vi "zmq proxy.vi"(8 "error in (no error)":errorcluster, 9 "capture_":u32, 10 "backend_":u32, 11 "frontend_":u32) -> (0 "error out":errorcluster, 1 "capture_ out":u32, 2 "backend_ out":u32, 3 "frontend_ out":u32, 5 "function return":i32)   [LabVIEW 2025, in "libzmq-v143-mt-4_3_6.lvlib"]
doc: "ZMQ_EXPORT int zmq_proxy (void *frontend_, void *backend_, void *capture_);"
uses:
  libzmq-v143-mt-4_3_6.lvlib
  LV/LibZMQ/libzmq/lv_x86/bin/Release/libzmq-v143-mt-4_3_6.dll
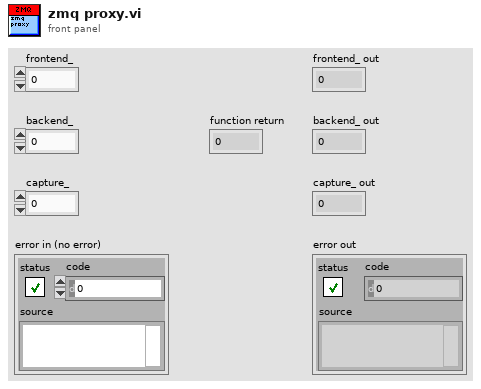
[diagram p1: front panel]
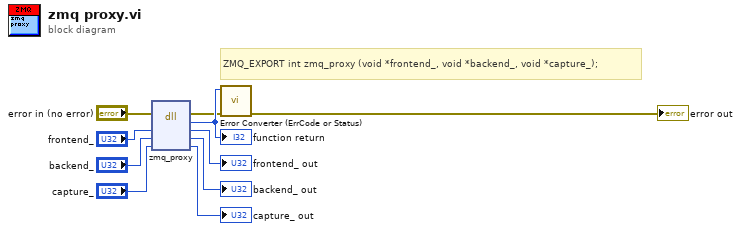
[diagram p0: block diagram]
diagram:
  # "ZMQ_EXPORT int zmq_proxy (void *frontend_, void *backend_, void *capture_);"
  n1 = dll-call lib="C:/LV/LibZMQ/libzmq/lv_x86/bin/Release/libzmq-v143-mt-4_3_6.*" fn="zmq_proxy"(error in="error in (no error)", "frontend_"="frontend_", "backend_"="backend_", "capture_"="capture_") -> (error out=w2:errorcluster, w10:i32, "frontend_"=→"frontend_ out":u32, "backend_"=→"backend_ out":u32, "capture_"=→"capture_ out":u32)  [unwired: 2 in, 1 out]
  "function return" <- w10
  n2 = call "Error Converter (ErrCode or Status).vi"("error in (no error)"=w2, "error code"=w10) -> ("error out"=→"error out":errorcluster)  [unwired: 9 in]
